vi "bronkhorst_reg_simple_ext.vi"(0 "SP":dbl caption="setpoint" step=0.01 format="%.2f", 1 "PV":dbl step=0.01 format="%.2f", 2 "PV_State":T3, 3 "Y":dbl step=0.01 format="%.2f", 4 "Y_State":T3, 6 "Y_Set":T5={"Y_HSw"=1, "Y_HSetState"=enum."auto", "Y_ASetState"=enum."auto", "Y_DSetState"=enum."auto"} {"Y_HSw" max=2 step=1}, 7 "controls Y":cluster{"Y_H":dbl, "Y_A":dbl, "Y_D":dbl} {"Y_H" format="%.2f"; "Y_D" format="%#_13g"; "Y_A" format="%#_13g"}, 8 "Z":T6, 9 "control param":T9={"output high"=1.0, "alr value"=10.0, "output low"=1.0, "output time (t)"=100.0} {"output time (t)" min=0.001 format="%.2f"; "output low" format="%.2f"; "alr value" format="%.2f"; "output high" format="%.2f"}, 10 "XB24 (F)":bool, 11 "Y_limiter_old":T1 {"output" format="%.2f"}, 12 "Start":bool) -> (13 "Y_limiter":T1 {"output" format="%.2f"}, 14 "Y_State":T7={"Y_Source"=enum."local disabled", "Y_SetState"=enum."auto", "SP_Set"=0.0, "SP"=0.0, "PV"=0.0, "PV_State"={"code"=0, "visible"=FALSE, "color"=0}, "Y_preSet"=0.0, "Y_Set"=0.0, "Y"=0.0, "Y_State"={"code"=0, "visible"=FALSE, "color"=0}, "YB"=FALSE} {"Y" format="%.2f"; "Y_preSet" format="%.2f"; "SP" step=0.01 format="%.2f"; "Y_Set" format="%.2f"; "PV" step=0.01 format="%.2f"; "SP_Set" step=0.01 format="%.2f"}, 15 "Y":dbl format="%.2f", 17 "T":u32, 18 "End":bool)   [LabVIEW 2019, in "control.lvlib"]
uses:
  control.lvlib
  ctl/control param simple.ctl
  ctl/Y.ctl
  ctl/Y_source.ctl
  ctl/Y_state.ctl
  Inputs/Ctl/Parameter State short.ctl
  ctl/Z_State.ctl
  ctl/Y_Lim_State.ctl
  ctl/Y_Lim_ext_defs.ctl
  PID/PID Output Rate Limiter Ext.vi
  PID/PID Timing Estimation Ext.vi
  Inputs/Inputs.lvlib
panel:
  out "SpLim_State":T2=enum."increase"
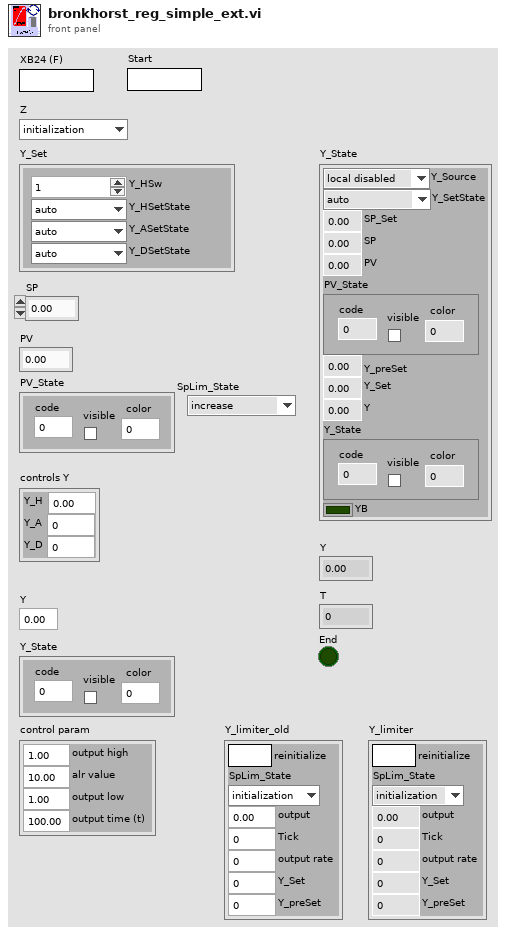
[diagram p1: front panel]
types:
  T1 = typedef "control.lvlib/Y_Lim_ext_defs.ctl" = cluster{"reinitialize":bool, "SpLim_State":T2, "output":dbl, "Tick":u32, "output rate":dbl, "Y_Set":dbl, "Y_preSet":dbl}
  T2 = typedef "control.lvlib/Y_Lim_State.ctl" = enum8{"initialization", "alarm", "stop", "decrease", "increase"}
  T3 = typedef "Inputs.lvlib/Parameter State short.ctl" = cluster{"code":i32, "visible":bool, "color":u32}
  T4 = typedef "control.lvlib/Y_state.ctl" = enum8{"initialize", "alarm", "min", "stop", "hand", "auto", "max"}
  T5 = cluster{"Y_HSw":u32, "Y_HSetState":T4, "Y_ASetState":T4, "Y_DSetState":T4}
  T6 = typedef "control.lvlib/Z_State.ctl" = enum8{"initialization", "alarm", "disabled", "not ready", "stop ready", "reserv", "switched off", "reserv2", "switched on", "check", "on min", "decrease out", "on", "increase out", "on max"}
  T7 = typedef "control.lvlib/Y.ctl" = cluster{"Y_Source":T8, "Y_SetState":T4, "SP_Set":dbl, "SP":dbl, "PV":dbl, "PV_State":T3, "Y_preSet":dbl, "Y_Set":dbl, "Y":dbl, "Y_State":T3, "YB":bool}
  T8 = typedef "control.lvlib/Y_source.ctl" = enum8{"initialize", "local disabled", "local hand", "hand", "auto", "dist"}
  T9 = typedef "control.lvlib/control param simple.ctl" = cluster{"output high":dbl, "alr value":dbl, "output low":dbl, "output time (t)":dbl}
  T10 = enum8{"alarm", "min", "stop", "hand", "auto", "max"}
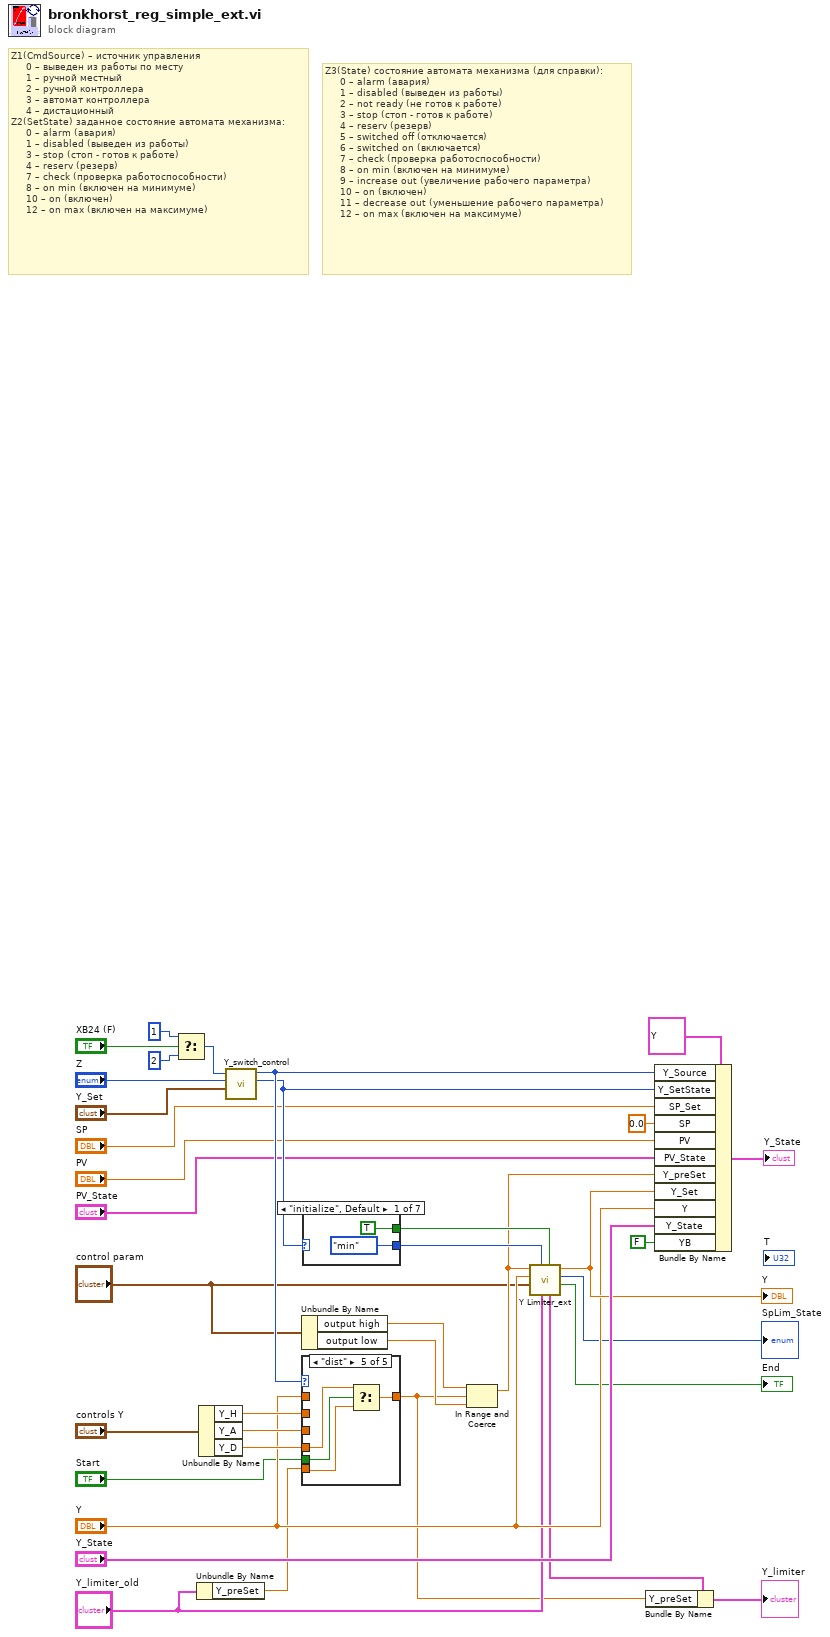
[diagram p0: block diagram]
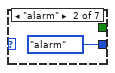
[diagram p2: hidden frame]
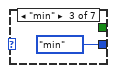
[diagram p3: hidden frame]
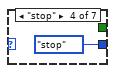
[diagram p4: hidden frame]
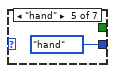
[diagram p5: hidden frame]
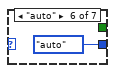
[diagram p6: hidden frame]
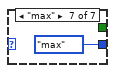
[diagram p7: hidden frame]
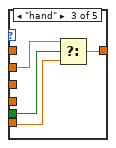
[diagram p10: hidden frame]
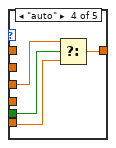
[diagram p11: hidden frame]
diagram:
  # "Z1(CmdSource) – источник управления\n     0 – выведен из работы по месту\n     1 – ручной местный\n     2 – ручной контроллера\n     3 – автомат контроллера\n     4 – дистационный\nZ2(SetState) заданное состояние автомата механизма:\n     0 – alarm (авария)\n     1 – disabled (выведен из работы)\n     3 – stop (стоп - готов к работе)\n     4 – reserv (резерв)\n     7 – check (проверка работоспособности)\n     8 – on min (включен на минимуме)\n     10 – on (включен)\n     12 – on max (включен на максимуме)"
  # "Z3(State) состояние автомата механизма (для справки):\n     0 – alarm (авария)\n     1 – disabled (выведен из работы)\n     2 – not ready (не готов к работе)\n     3 – stop (стоп - готов к работе)\n     4 – reserv (резерв)\n     5 – switched off (отключается)\n     6 – switched on (включается)\n     7 – check (проверка работоспособности)\n     8 – on min (включен на минимуме)\n     9 – increase out (увеличение рабочего параметра)\n     10 – on (включен)\n     11 – decrease out (уменьшение рабочего параметра)\n     12 – on max (включен на максимуме)"
  n1 = Select(t=u32 1, s="XB24 (F)", f=u32 2 ("Y_HSw")) -> (s? t:f=w32:u32)
  n2 = Unbundle By Name("Y_limiter_old") -> ("Y_preSet"=w6:dbl)
  n3 = Unbundle By Name("controls Y") -> ("Y_H"=w20:dbl, "Y_A"=w36:dbl, "Y_D"=w35:dbl)
  n4 = call "Y_switch_control.vi"("Y"="Y_Set", "Z_State"="Z", "Y_LSw (2-auto)"=w32) -> ("Y_SetState"=w29:T4, "Y_Source"=w30:T8)  [unwired: 7 in]
  n5 = Unbundle By Name("control param") -> ("output high"=w12:dbl, "output low"=w10:dbl)
  n6 = case shown="\"dist\"" w30 {
    tunnel: w20 -> [_ _ w39 _ _]
    tunnel: "Y" -> [w37 w38 _ _ _]
    tunnel: w35 -> [_ _ _ _ w49]
    tunnel: [w37 w38 w42 w46 w50] -> w2
    tunnel: w36 -> [_ _ _ w43 _]
    tunnel: w6 -> [_ _ w41 w45 w48]
    tunnel: "Start" -> [_ _ w40 w44 w47]
    frame "local disabled", Default {
    }
    frame "local hand" {
    }
    frame "hand" {
      n7 = Select(t=w39, s=w40, f=w41) -> (s? t:f=w42:dbl)
    }
    frame "auto" {
      n8 = Select(t=w43, s=w44, f=w45) -> (s? t:f=w46:dbl)
    }
    frame "dist" {
      n9 = Select(t=w49, s=w47, f=w48) -> (s? t:f=w50:dbl)
    }
  }
  n10 = case shown="\"initialize\", Default" w29 {
    tunnel: [T10."min" ("X1(SetState)") T10."alarm" ("X1(SetState)") T10."min" ("X1(SetState)") T10."stop" ("X1(SetState)") T10."hand" ("X1(SetState)") T10."auto" ("X1(SetState)") T10."max" ("X1(SetState)")] -> w16
    tunnel: [TRUE _ _ _ _ _ _] -> w18
    frame "initialize", Default {
    }
    frame "alarm" {
    }
    frame "min" {
    }
    frame "stop" {
    }
    frame "hand" {
    }
    frame "auto" {
    }
    frame "max" {
    }
  }
  n11 = In Range and Coerce(upper limit=w12, x=w2, lower limit=w10) -> (coerced(x)=w11:dbl)  [unwired: 1 out]
  n12 = call "Y Limiter_ext.vi"("reinitialize? (F)"=w18, "Y_limiter_old"="Y_limiter_old", "X1(SetState)"=w16, "Y param"="control param", "Y (NaN)"="Y", "Y_Set"=w11) -> ("End"=→"End":bool, "SpLim_State"=→"SpLim_State":T2, "output"=w19:dbl, "Y_limiter"=w4:T1)  [unwired: 2 in]
  "Y" <- w19
  n13 = Bundle By Name(cluster=w4, "Y_preSet"=w2) -> (→"Y_limiter":T1)
  n14 = Bundle By Name(cluster=T7 {"Y_Source"=enum."local disabled", "Y_SetState"=enum."auto", "SP_Set"=0.0, "SP"=0.0, "PV"=0.0, "PV_State"={"code"=0, "visible"=FALSE, "color"=0}, "Y_preSet"=0.0, "Y_Set"=0.0, "Y"=0.0, "Y_State"={"code"=0, "visible"=FALSE, "color"=0}, "YB"=FALSE} ("Y_State"), "Y_Source"=w30, "Y_SetState"=w29, "SP_Set"="SP", "SP"=0.0, "PV"="PV", "PV_State"="PV_State", "Y_preSet"=w11, "Y_Set"=w19, "Y"="Y", "Y_State"="Y_State", "YB"=FALSE) -> (→"Y_State":T7)
